vi "PC main.vi"() -> ()   [LabVIEW 2017]
uses:
  <vilib>/FPGAPlugInAG/cRIO-9065/niLvFpga_Open_cRIO-9065.vi
  <vilib>/rvi/interface/common/dynamic/niFpgaDynamicAddResources.vi
  <vilib>/Utility/error.llb/Error Cluster From Error Code.vi
  <vilib>/rvi/errors/niLvFpgaAdjustHostInterfaceError.vi
  <vilib>/FPGAPlugInAG/Dynamic/niLvFpga_Run_Dynamic.vi
  <vilib>/FPGAPlugInAG/Dynamic/niLvFpga_Abort_Dynamic.vi
  <vilib>/rvi/interface/nirviOpenFPGA/nirviOpenFPGA.xnode
  FPGA Bitfiles/fpgaproject_FPGATarget_fpgamain2_gPNnZPUgBMY.lvbitx
  fpga main2.vi
  <vilib>/rvi/interface/nirviMethod/nirviMethod.xnode
  <vilib>/rvi/interface/nirviReadWriteControl/nirviReadWriteControl.xnode
  NiFpgaLv.dll
  <vilib>/rvi/interface/Simulation/niFpgaSimulationCallBeginRW.vi
  <vilib>/FPGAPlugInAG/Dynamic/niLvFpga_StartFifo_Dynamic.vi
  <vilib>/rvi/errors/niLvFpgaMergeErrorWithErrorCode.vi
  <vilib>/FPGAPlugInAG/Dynamic/niLvFpga_ReadFifo_Dynamic.vi
panel:
  out "x-y":u32
  out "error out 3":errorcluster
  in  "stop":bool
  out "Data":i16[](array[numeric])
  out "error out 2":errorcluster
  in  "Velocity Interval (uSec)":u32
  out "error out":errorcluster
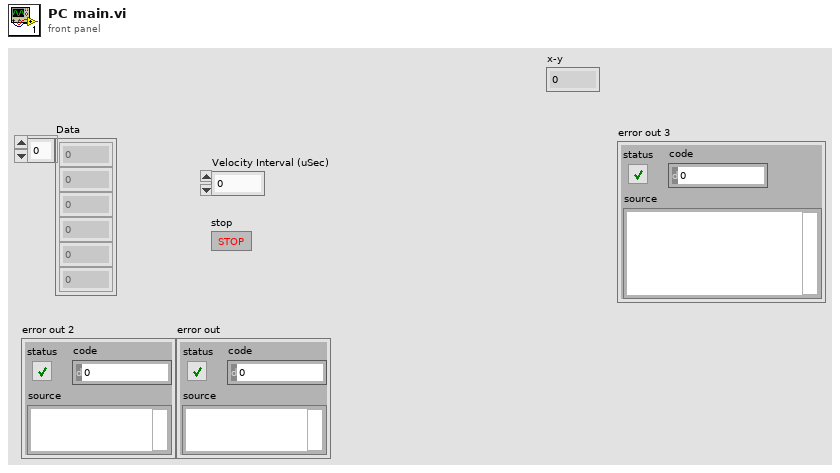
[diagram p1: front panel]
types:
  T1 = enum16{"open", "replace", "create", "open or create", "replace or create", "replace or create with confirmation"}
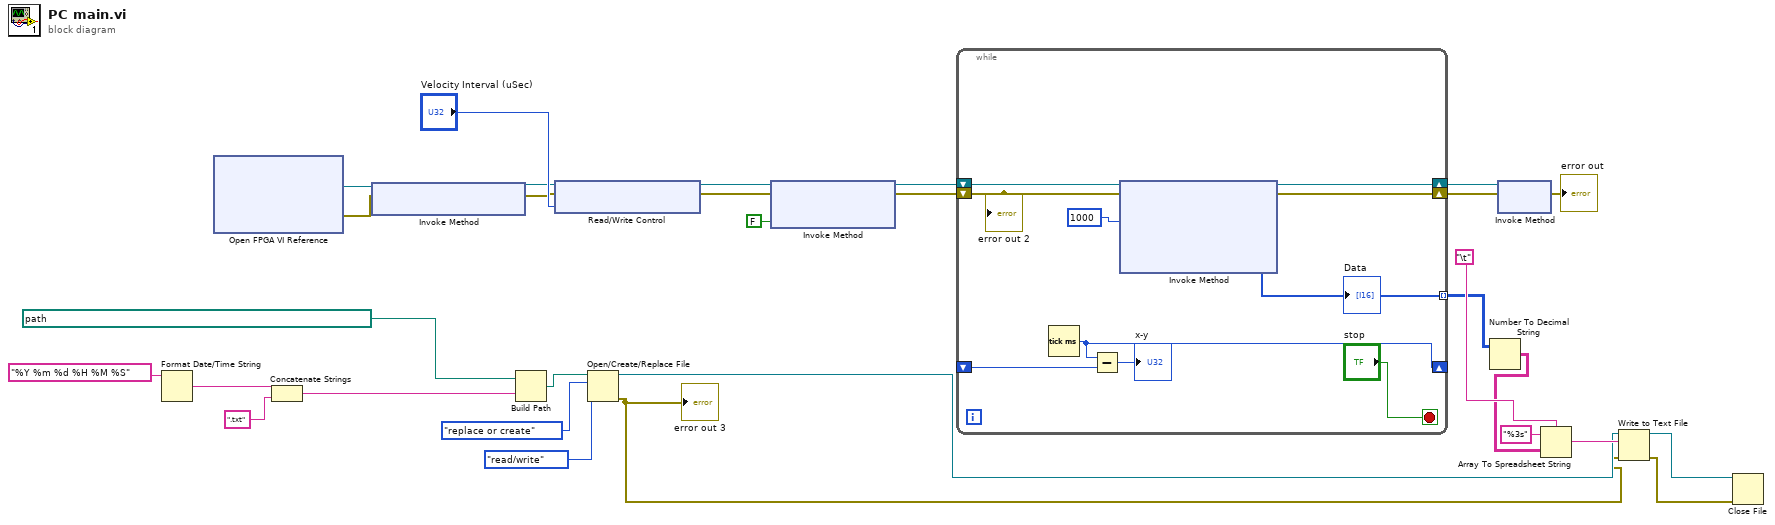
[diagram p0: block diagram]
diagram:
  n1 = Format Date/Time String(time format string (%c)="%Y %m %d %H %M %S") -> (date/time string=w16:string)  [unwired: 2 in]
  n2 = xnode "Open FPGA VI Reference"() -> ("FPGA VI Reference Out"=w19:refnum<k20>, "error out"=w18:errorcluster)  [unwired: 2 in]
  n3 = Concatenate Strings(w16, ".txt" ("string")) -> (w14:string)
  n4 = xnode "Invoke Method"("FPGA VI Reference In"=w19, "error in"=w18) -> ("FPGA VI Reference Out"=w22:refnum<k20>, "error out"=w21:errorcluster)
  n5 = Build Path(base path=path "\\\\LAPTOP-RMK8J9U6\\Users/baby3/Desktop/fpga/數據儲存", name or relative path=w14) -> (appended path=w12:path)
  n6 = xnode "Read/Write Control"("FPGA VI Reference In"=w22, "error in"=w21, "Velocity Interval (uSec)"="Velocity Interval (uSec)") -> ("FPGA VI Reference Out"=w25:refnum<k20>, "error out"=w24:errorcluster)
  n7 = Open/Create/Replace File(file path (use dialog)=w12, operation (0:open)=T1."replace or create", access (0:read/write)=enum16{"read/write", "read-only", "write-only"}."read/write") -> (refnum out=w5:refnum<file>, error out=w4:errorcluster)  [unwired: 3 in, 1 out]
  "error out 3" <- w4
  n8 = xnode "Invoke Method"("FPGA VI Reference In"=w25, "error in"=w24, "Wait Until Done (F)"=FALSE) -> ("FPGA VI Reference Out"=w27:refnum<k20>, "error out"=w26:errorcluster)
  n9 = while {
    shift-right: [w40] -> w30
    shift-left: w27 -> [w38]
    shift-right: [w39] -> w29
    shift-left: w26 -> [w37]
    tunnel: [w34] -> w9 mode=indexing
    shift-right: [w32] -> _
    shift-left: _ -> [w33]
    stop <- "stop" stop-if-true
    n10 = Tick Count (ms)() -> (millisecond timer value=w32:u32)
    n11 = Subtract(x=w32, y=w33) -> (x-y=→"x-y":u32)
    n12 = xnode "Invoke Method"("FPGA VI Reference In"=w38, "error in"=w37, "Number of Elements"=u32 1000) -> ("FPGA VI Reference Out"=w40:refnum<k20>, "error out"=w39:errorcluster, "Data"=w34:i16[])  [unwired: 1 in, 1 out]
    "Data" <- w34
    "error out 2" <- w37
  }
  n13 = Number To Decimal String(number=w9) -> (decimal integer string=w8:string[][])  [unwired: 1 in]
  n14 = xnode "Invoke Method"("FPGA VI Reference In"=w30, "error in"=w29) -> ("error out"=→"error out":errorcluster)  [unwired: 1 out]
  n15 = Array To Spreadsheet String(delimiter (Tab)="\t", array=w8, 3:"%3s" ("format string")) -> (spreadsheet string=w6:string)
  n16 = Write to Text File(file (use dialog)=w5, text=w6, error in=w4) -> (refnum out=w2:refnum<file>, error out=w3:errorcluster)  [unwired: 1 in, 1 out]
  n17 = Close File(refnum=w2, error in=w3) -> ()  [unwired: 2 out]
